vi "setBoardID.vi"(8 "error in (no error)":errorcluster, 10 "boardID":i32, 11 "Pixelfly in":refnum<class "PixelflySA.lvclass">) -> (0 "error out":errorcluster, 3 "Pixelfly out":refnum<class "PixelflySA.lvclass">)   [LabVIEW 2011, in "PixelflySA.lvclass"]
uses:
  PixelflySA.lvclass
  PixelflySA.lvclass/PixelflySA.ctl
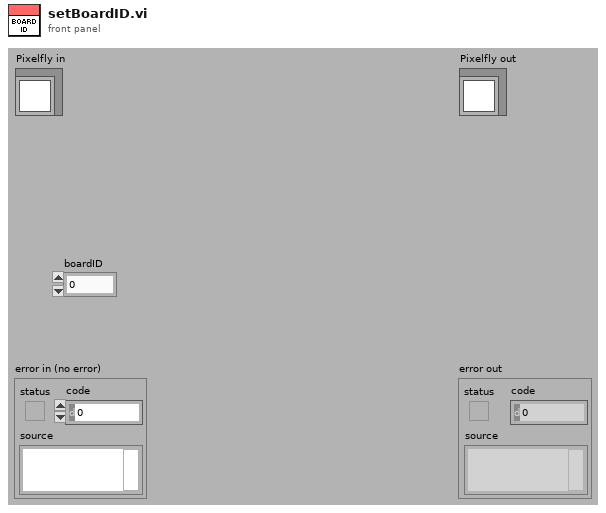
[diagram p1: front panel]
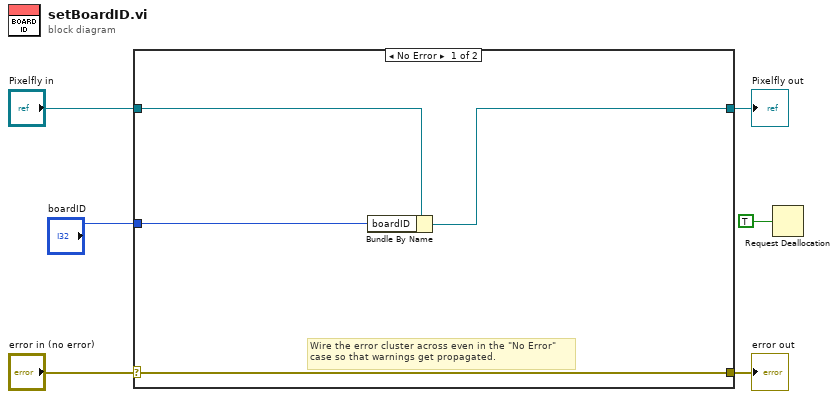
[diagram p0: block diagram]
diagram:
  n1 = case shown="No Error" "error in (no error)" {
    selector: "error in (no error)" -> [w10 w12]
    tunnel: [w10 w12] -> w5
    tunnel: [w7 w11] -> w3
    tunnel: "Pixelfly in" -> [w8 w11]
    tunnel: "boardID" -> [w9 _]
    frame No Error {
      # "Wire the error cluster across even in the \"No Error\"\ncase so that warnings get propagated."
      n2 = Bundle By Name(cluster=w8, "boardID"=w9) -> (w7:refnum<class "PixelflySA.lvclass">)
    }
    frame Error {
    }
  }
  "error out" <- w5
  "Pixelfly out" <- w3
  n3 = Request Deallocation(TRUE ("flag")) -> ()
